vi "controlReferenceAutoUpdate.vi"(7 "Set":bool, 8 "error in":errorcluster, 9 "Enable":bool, 10 "axis in":u8, 11 "connection ID":refnum<k5>) -> (0 "error out":errorcluster, 1 "Enable Out":bool, 2 "axis out":i32, 3 "connection ID":refnum<k5>)   [LabVIEW 2016, in "AMC_VIs.lvlib"]
doc: "This function retrieves or sets the status of whether the reference position is updated when the reference mark is hit."
uses:
  AMC_VIs.lvlib
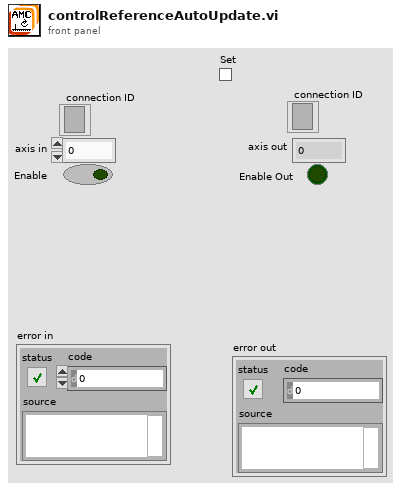
[diagram p1: front panel]
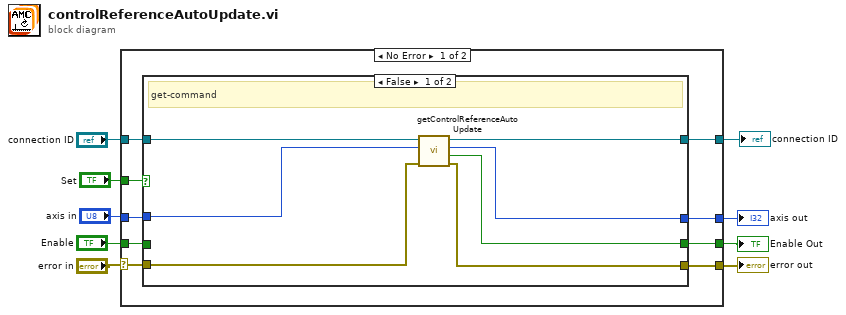
[diagram p0: block diagram]
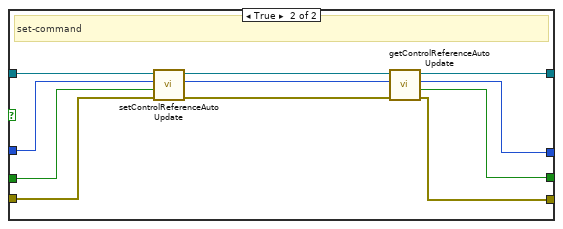
[diagram p2: hidden frame]
diagram:
  n1 = case shown="No Error" "error in" {
    selector: "error in" -> [w14 w40]
    tunnel: "axis in" -> [w18 w37]
    tunnel: [w12 w40] -> w8
    tunnel: "Enable" -> [w16 w38]
    tunnel: [w13 w38] -> w3
    tunnel: "Set" -> [w15 _]
    tunnel: [w10 w39] -> w6
    tunnel: "connection ID" -> [w17 w39]
    tunnel: [w11 w37] -> w1
    frame No Error {
      n2 = case shown="False" w15 {
        tunnel: w17 -> [w23 w36]
        tunnel: w18 -> [w22 w34]
        tunnel: w16 -> [_ w33]
        tunnel: w14 -> [w25 w32]
        tunnel: [w19 w27] -> w13
        tunnel: [w24 w29] -> w12
        tunnel: [w20 w28] -> w11
        tunnel: [w21 w26] -> w10
        frame False {
          # "get-command"
          n3 = call "getControlReferenceAutoUpdate.vi"("error in"=w25, "axis"=w22, "connection ID"=w23) -> ("error out"=w24:errorcluster, "enabled"=w19:bool, "axis_out"=w20:i32, "connection ID"=w21:refnum<k5>)  [unwired: 5 in]
        }
        frame True {
          # "set-command"
          n4 = call "setControlReferenceAutoUpdate.vi"("error in"=w32, "enable"=w33, "axis"=w34, "connection ID"=w36) -> ("error out"=w31:errorcluster, "axis_out"=w30:i32, "connection ID"=w35:refnum<k5>)  [unwired: 5 in]
          n5 = call "getControlReferenceAutoUpdate.vi"("error in"=w31, "axis"=w30, "connection ID"=w35) -> ("error out"=w29:errorcluster, "enabled"=w27:bool, "axis_out"=w28:i32, "connection ID"=w26:refnum<k5>)  [unwired: 5 in]
        }
      }
    }
    frame Error {
    }
  }
  "error out" <- w8
  "axis out" <- w1
  "Enable Out" <- w3
  "connection ID" <- w6
